vi "TemperatureControl.vi"() -> ()   [LabVIEW 2015]
panel:
  in  "Low Value":dbl
  in  "High Value":dbl
  out "Waveform Chart":dbl(graph)
  out "Thermometer":dbl(slide) scale=0.0..50.0
  out "Temperature Value":dbl
  out "YLDRMErrorOut":errorcluster
  out "YLDRMPortOut":refnum<visa-resource-name>
  in  "YLDRMPortInp":refnum<visa-resource-name>
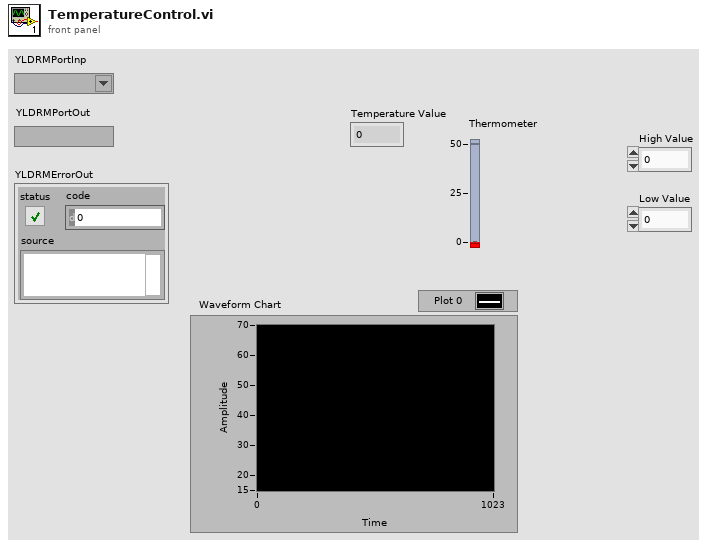
[diagram p1: front panel]
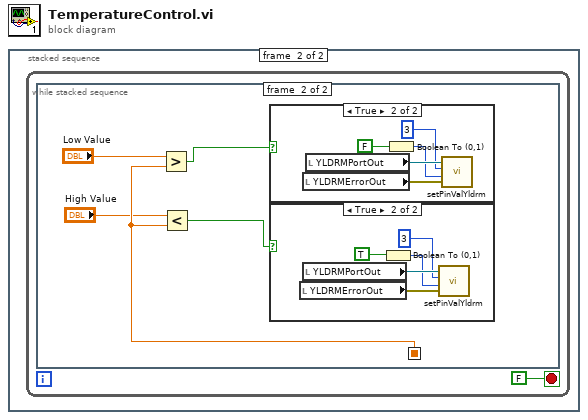
[diagram p0: block diagram]
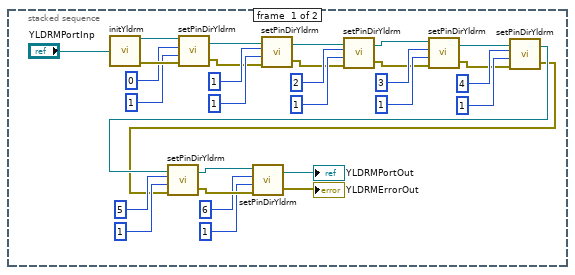
[diagram p2: hidden frame]
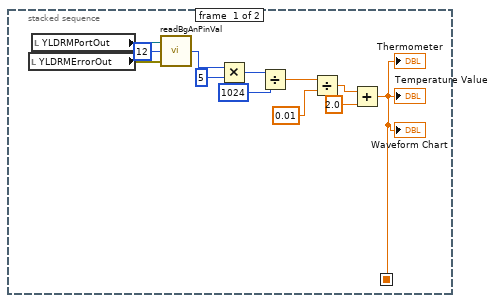
[diagram p3: hidden frame]
diagram:
  n1 = stacked-sequence {
    frame #0 {
      n2 = call "initYldrm.vi"("YLDRMPortInp"="YLDRMPortInp") -> ("YLDRMPortOut"=w30:refnum<visa-resource-name>, "YLDRMErrorOut"=w29:errorcluster)
      n3 = call "setPinDirYldrm.vi"("YLDRMErrorInp"=w29, "dir"=u8 1, "pin"=u8 0, "YLDRMPortInp"=w30) -> ("YLDRMErrorOut"=w17:errorcluster, "YLDRMPortOut"=w18:refnum<visa-resource-name>)
      n4 = call "setPinDirYldrm.vi"("YLDRMErrorInp"=w17, "dir"=u8 1, "pin"=u8 1, "YLDRMPortInp"=w18) -> ("YLDRMErrorOut"=w15:errorcluster, "YLDRMPortOut"=w16:refnum<visa-resource-name>)
      n5 = call "setPinDirYldrm.vi"("YLDRMErrorInp"=w15, "dir"=u8 1, "pin"=u8 2, "YLDRMPortInp"=w16) -> ("YLDRMErrorOut"=w13:errorcluster, "YLDRMPortOut"=w14:refnum<visa-resource-name>)
      n6 = call "setPinDirYldrm.vi"("YLDRMErrorInp"=w13, "dir"=u8 1, "pin"=u8 3, "YLDRMPortInp"=w14) -> ("YLDRMErrorOut"=w11:errorcluster, "YLDRMPortOut"=w12:refnum<visa-resource-name>)
      n7 = call "setPinDirYldrm.vi"("YLDRMErrorInp"=w11, "dir"=u8 1, "pin"=u8 4, "YLDRMPortInp"=w12) -> ("YLDRMErrorOut"=w3:errorcluster, "YLDRMPortOut"=w4:refnum<visa-resource-name>)
      n8 = call "setPinDirYldrm.vi"("YLDRMErrorInp"=w3, "dir"=u8 1, "pin"=u8 5, "YLDRMPortInp"=w4) -> ("YLDRMErrorOut"=w10:errorcluster, "YLDRMPortOut"=w9:refnum<visa-resource-name>)
      n9 = call "setPinDirYldrm.vi"("YLDRMErrorInp"=w10, "dir"=u8 1, "pin"=u8 6, "YLDRMPortInp"=w9) -> ("YLDRMErrorOut"=→"YLDRMErrorOut":errorcluster, "YLDRMPortOut"=→"YLDRMPortOut":refnum<visa-resource-name>)
    }
    frame #1 {
      n10 = while {
        stop <- FALSE stop-if-true
        n11 = stacked-sequence {
          seq-local: [w33 _] -> [_ w49]
          frame #0 {
            n12 = local read "YLDRMErrorOut"() -> (w43:errorcluster)
            n13 = local read "YLDRMPortOut"() -> (w44:refnum<visa-resource-name>)
            n14 = call "readBgAnPinVal.vi"("YLDRMErrorInp"=w43, "pin"=u8 12, "YLDRMPortInp"=w44) -> ("out"=w41:u16)  [unwired: 2 out]
            n15 = Multiply(x=w41, y=u16 5) -> (x*y=w39:u16)
            n16 = Divide(x=w39, y=u16 1024) -> (x/y=w37:dbl)
            n17 = Divide(x=w37, y=0.01) -> (x/y=w35:dbl)
            n18 = Add(x=w35, y=2.0) -> (x+y=w33:dbl)
            "Temperature Value" <- w33
            "Waveform Chart" <- w33
            "Thermometer" <- w33
          }
          frame #1 {
            n19 = Greater?(x="Low Value", y=w49) -> (0:w46:bool)
            n20 = Less?(x="High Value", y=w49) -> (x < y?=w45:bool)
            n21 = case shown="True" w46 {
              frame False {
              }
              frame True {
                n22 = local read "YLDRMErrorOut"() -> (w53:errorcluster)
                n23 = local read "YLDRMPortOut"() -> (w54:refnum<visa-resource-name>)
                n24 = Boolean To (0,1)(Boolean=FALSE) -> (0, 1=w51:i16)
                n25 = call "setPinValYldrm.vi"("YLDRMErrorInp"=w53, "val"=w51, "pin"=3, "YLDRMPortInp"=w54) -> ()  [unwired: 2 out]
              }
            }
            n26 = case shown="True" w45 {
              frame False {
              }
              frame True {
                n27 = local read "YLDRMErrorOut"() -> (w58:errorcluster)
                n28 = local read "YLDRMPortOut"() -> (w59:refnum<visa-resource-name>)
                n29 = Boolean To (0,1)(Boolean=TRUE) -> (0, 1=w56:i16)
                n30 = call "setPinValYldrm.vi"("YLDRMErrorInp"=w58, "val"=w56, "pin"=3, "YLDRMPortInp"=w59) -> ()  [unwired: 2 out]
              }
            }
          }
        }
      }
    }
  }
